vi "di_oneshot_full.vi"() -> ()   [LabVIEW 2020]
uses:
  <vilib>/Waveform/DWDTOps.llb/DWDT Analog to Digital.vi
panel:
  out "error out":errorcluster caption="错误输出"
  out "数字波形图":digitalwaveform(graph)
  in  "DiOneShotPoints":u32=1000
  in  "SamplePeriod":u32=10000 caption="SamplePeriod (ns)"
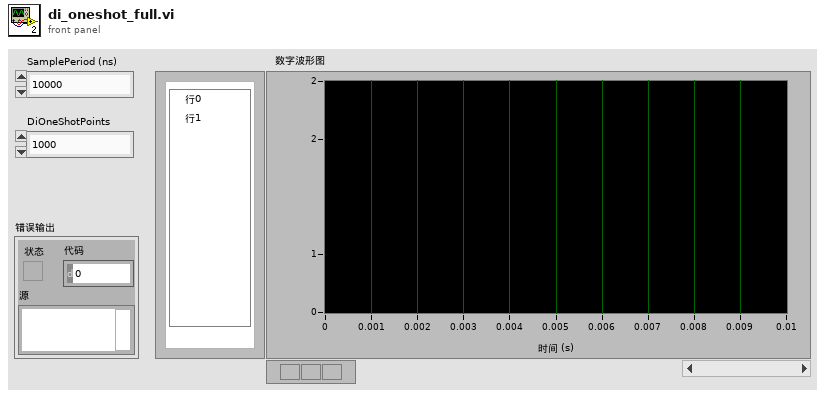
[diagram p1: front panel]
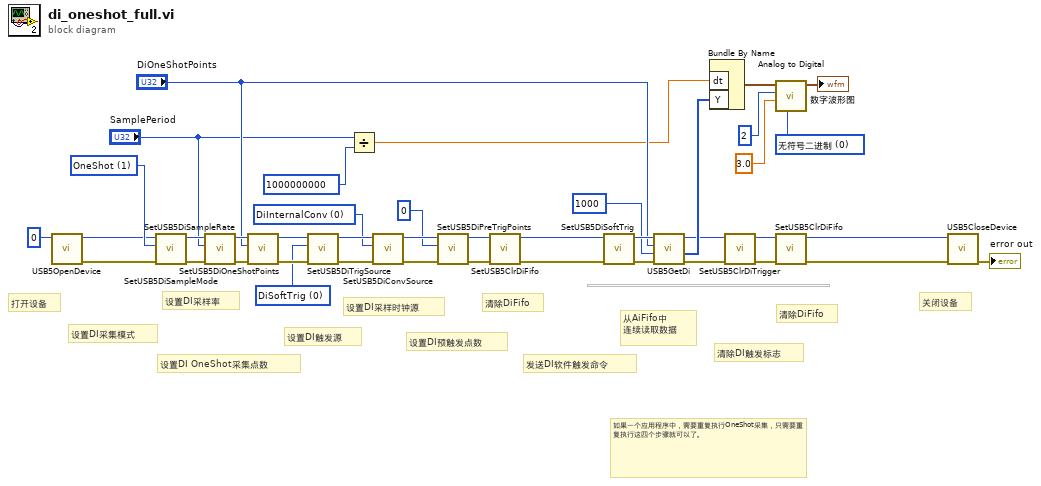
[diagram p0: block diagram]
diagram:
  w1 = u8 0 items=["DiInternalConv"=0, "ConvIn"=1, "AiConv"=2, "DoConv"=4, "Ao0Conv"=5, "Ao1Conv"=6, "Ao2Conv"=7, "Ao3Conv"=8] ("DiConvSource")
  w2 = u8 0 items=["DiSoftTrig"=0, "ExtTrigIn"=1, "Din0RisingEdge"=2, "Din1RisingEdge"=3, "Din2RisingEdge"=4, "Din3RisingEdge"=5, "WithAiTrig"=6, "WithDoTrig"=8, "WithAo0Trig"=9, "WithAo1Trig"=10, "WithAo2Trig"=11, "WithAo3Trig"=12, "GlobalSoftTrig"=255] ("DiTrigSource")
  w26 = u16 0 items=["无符号二进制", "二进制偏移量", "二进制补码"] ("data format (offset binary)")
  w40 = u8 1 items=["Continuous", "OneShot"] ("DiSampleMode")
  # "如果一个应用程序中，需要重复执行OneShot采集，只需要重复执行这四个步骤就可以了。"
  # "关闭设备"
  # "清除DiFifo"
  # "清除DI触发标志"
  # "从AiFifo中\n连续读取数据"
  # "发送DI软件触发命令"
  # "清除DiFifo"
  # "设置DI预触发点数"
  # "设置DI采样时钟源"
  # "设置DI触发源"
  # "设置DI OneShot采集点数"
  # "设置DI采样率"
  # "设置DI采集模式"
  # "打开设备"
  n1 = call "USB5OpenDevice.vi"("DevIndex"=0) -> ("error out"=w4:errorcluster, "DevIndex Out"=w5:i32)  [unwired: 9 in]
  n2 = call "SetUSB5DiSampleMode.vi"("错误输入（无错误）"=w4, "DiSampleMode"=w40, "DevIndex"=w5) -> ("错误输出"=w39:errorcluster, "DevIndex Out"=w38:i32)  [unwired: 7 in]
  n3 = call "SetUSB5DiSampleRate.vi"("错误输入（无错误）"=w39, "SamplePeriod(ns)"="SamplePeriod", "DevIndex"=w38) -> ("错误输出"=w37:errorcluster, "DevIndex Out"=w36:i32)  [unwired: 7 in]
  n4 = call "SetUSB5DiOneShotPoints.vi"("错误输入（无错误）"=w37, "DiOneShotPoints"="DiOneShotPoints", "DevIndex"=w36) -> ("错误输出"=w15:errorcluster, "DevIndex Out"=w16:i32)  [unwired: 7 in]
  n5 = call "SetUSB5DiTrigSource.vi"("错误输入（无错误）"=w15, "DiTrigSource"=w2, "DevIndex"=w16) -> ("错误输出"=w12:errorcluster, "DevIndex Out"=w14:i32)  [unwired: 7 in]
  n6 = Divide(x="SamplePeriod", y=u32 1000000000) -> (x/y=w23:dbl)
  n7 = call "SetUSB5DiConvSource.vi"("错误输入（无错误）"=w12, "DiConvSource"=w1, "DevIndex"=w14) -> ("错误输出"=w11:errorcluster, "DevIndex Out"=w13:i32)  [unwired: 7 in]
  n8 = call "SetUSB5DiPreTrigPoints.vi"("错误输入（无错误）"=w11, "DiPreTrigPoints"=u32 0, "DevIndex"=w13) -> ("错误输出"=w8:errorcluster, "DevIndex Out"=w9:i32)  [unwired: 7 in]
  n9 = call "SetUSB5ClrDiFifo.vi"("错误输入（无错误）"=w8, "DevIndex"=w9) -> ("错误输出"=w6:errorcluster, "DevIndex Out"=w7:i32)  [unwired: 8 in]
  n10 = call "SetUSB5DiSoftTrig.vi"("错误输入（无错误）"=w6, "DevIndex"=w7) -> ("错误输出"=w34:errorcluster, "DevIndex Out"=w35:i32)  [unwired: 8 in]
  n11 = call "USB5GetDi.vi"("错误输入（无错误）"=w34, "TimeOut"=1000, "Points"="DiOneShotPoints", "DevIndex"=w35) -> ("错误输出"=w18:errorcluster, "Di"=w22:u8[], "DevIndex Out"=w19:i32)  [unwired: 4 in, 1 out]
  n12 = Bundle By Name("dt"=w23, "Y"=w22) -> (w25:waveform(u8))  [unwired: 1 in]
  n13 = call "SetUSB5ClrDiTrigger.vi"("错误输入（无错误）"=w18, "DevIndex"=w19) -> ("错误输出"=w21:errorcluster, "DevIndex Out"=w20:i32)  [unwired: 8 in]
  n14 = call-poly <vilib>:"Analog to Digital.vi"("data format (offset binary)"=w26, "full-scale range (pk-pk)"=3.0, "resolution (16 bit)"=2, "analog waveform"=w25) -> ("digital waveform"=→"数字波形图":digitalwaveform)  [unwired: 4 in, 3 out]
  n15 = call "SetUSB5ClrDiFifo.vi"("错误输入（无错误）"=w21, "DevIndex"=w20) -> ("错误输出"=w29:errorcluster, "DevIndex Out"=w30:i32)  [unwired: 8 in]
  n16 = call "USB5CloseDevice.vi"("错误输入（无错误）"=w29, "DevIndex"=w30) -> ("error out"=→"error out":errorcluster)  [unwired: 8 in, 1 out]
